vi "Get Safety Enclosure Position.vi"(8 "error in (no error)":errorcluster, 11 "ESM303 in":refnum<class "ESM303.lvclass">) -> (0 "error out":errorcluster, 2 "Position (Closed = TRUE)":bool, 3 "ESM303 out":refnum<class "ESM303.lvclass">)   [LabVIEW 2018, in "ESM303.lvlib" / "ESM303.lvclass"]
uses:
  ESM303.lvclass
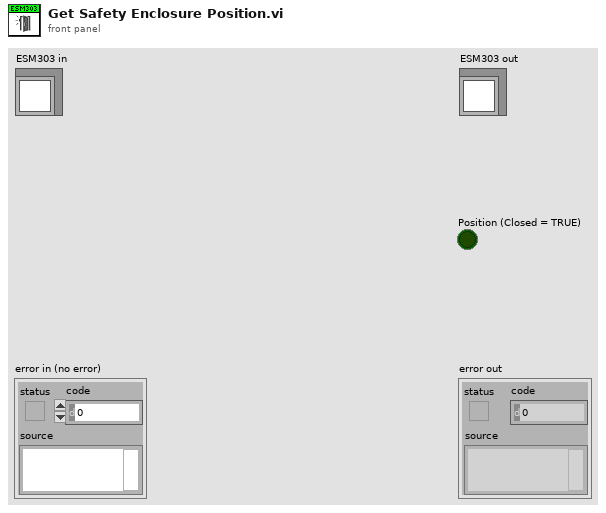
[diagram p1: front panel]
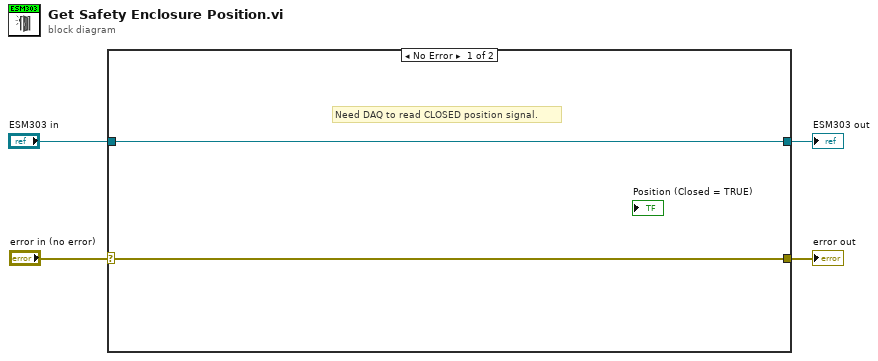
[diagram p0: block diagram]
diagram:
  n1 = case shown="No Error" "error in (no error)" {
    selector: "error in (no error)" -> [w5 w8]
    tunnel: [w5 w8] -> w3
    tunnel: [w6 w7] -> w2
    tunnel: "ESM303 in" -> [w6 w7]
    frame No Error {
      # "Need DAQ to read CLOSED position signal."
    }
    frame Error {
    }
  }
  "error out" <- w3
  "ESM303 out" <- w2
